vi "MGCC_MdlMgmt_others.vi"() -> ()   [LabVIEW 2016]
doc: "This VI is designed to initize the SHE215 model with Slack, NumN, NumL, NumC, NumZ, NumR and NumS (double)."
panel:
  out "text":string
  out "array":dbl[](array[numeric])
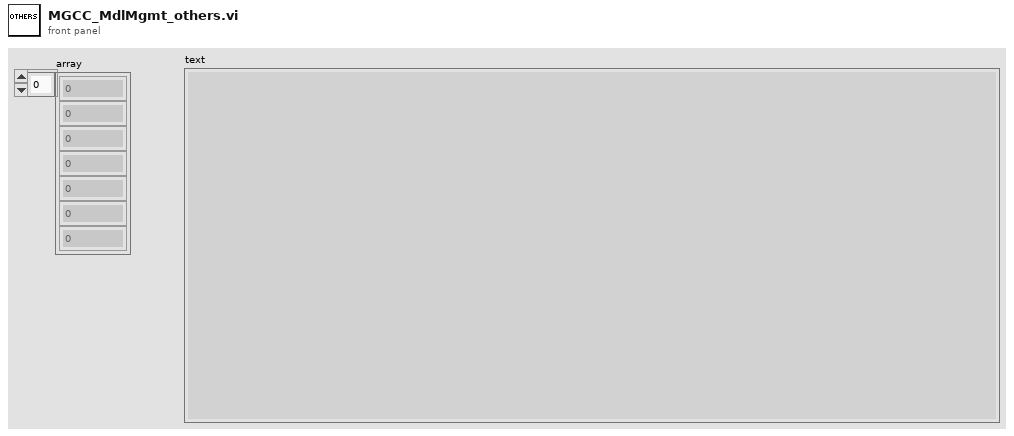
[diagram p1: front panel]
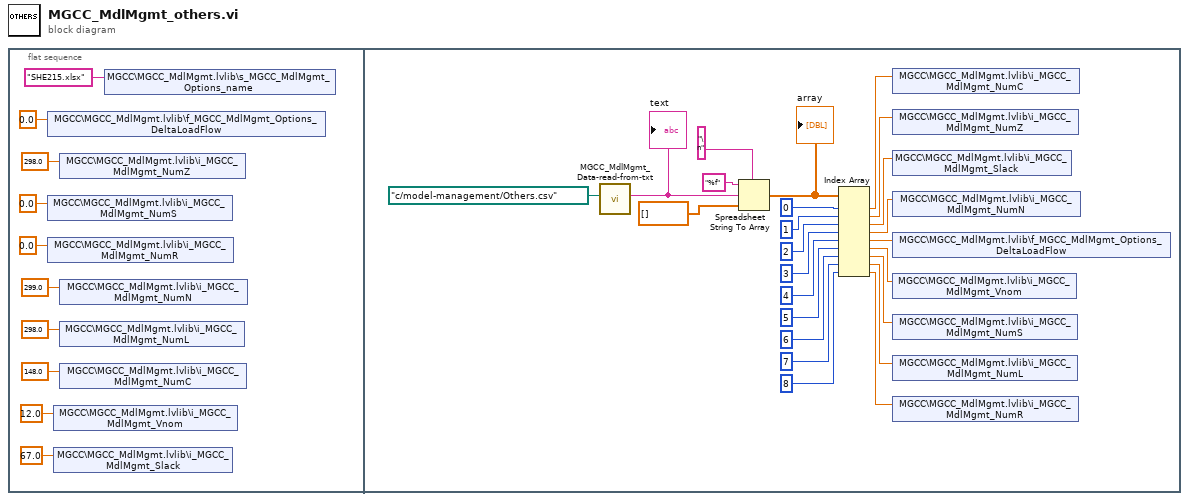
[diagram p0: block diagram]
diagram:
  n1 = flat-sequence {
    frame #0 {
      n2 = shared-variable "MGCC\\MGCC_MdlMgmt.lvlib\\f_MGCC_MdlMgmt_Options_DeltaLoadFlow"(0.0 ("MGCC_MdlMgmt_Options_DeltaLoadFlow")) -> ()  [unwired: 1 in, 1 out]
      n3 = shared-variable "MGCC\\MGCC_MdlMgmt.lvlib\\i_MGCC_MdlMgmt_NumS"(0.0 ("MGCC_MdlMgmt_NumS")) -> ()  [unwired: 1 in, 1 out]
      n4 = shared-variable "MGCC\\MGCC_MdlMgmt.lvlib\\i_MGCC_MdlMgmt_NumR"(0.0 ("MGCC_MdlMgmt_NumR")) -> ()  [unwired: 1 in, 1 out]
      n5 = shared-variable "MGCC\\MGCC_MdlMgmt.lvlib\\i_MGCC_MdlMgmt_Vnom"(12.0 ("MGCC_MdlMgmt_Vnom")) -> ()  [unwired: 1 in, 1 out]
      n6 = shared-variable "MGCC\\MGCC_MdlMgmt.lvlib\\i_MGCC_MdlMgmt_Slack"(67.0 ("MGCC_MdlMgmt_Slack")) -> ()  [unwired: 1 in, 1 out]
      n7 = shared-variable "MGCC\\MGCC_MdlMgmt.lvlib\\i_MGCC_MdlMgmt_NumZ"(298.0 ("MGCC_MdlMgmt_NumZ")) -> ()  [unwired: 1 in, 1 out]
      n8 = shared-variable "MGCC\\MGCC_MdlMgmt.lvlib\\i_MGCC_MdlMgmt_NumN"(299.0 ("MGCC_MdlMgmt_NumN")) -> ()  [unwired: 1 in, 1 out]
      n9 = shared-variable "MGCC\\MGCC_MdlMgmt.lvlib\\i_MGCC_MdlMgmt_NumL"(298.0 ("MGCC_MdlMgmt_NumL")) -> ()  [unwired: 1 in, 1 out]
      n10 = shared-variable "MGCC\\MGCC_MdlMgmt.lvlib\\i_MGCC_MdlMgmt_NumC"(148.0 ("MGCC_MdlMgmt_NumC")) -> ()  [unwired: 1 in, 1 out]
      n11 = shared-variable "MGCC\\MGCC_MdlMgmt.lvlib\\s_MGCC_MdlMgmt_Options_name"("SHE215.xlsx" ("MGCC_MdlMgmt_Options_name")) -> ()  [unwired: 1 in, 1 out]
    }
    frame #1 {
      n12 = call "MGCC_MdlMgmt_Data-read-from-txt.vi"("file path (use dialog)"=path "c:/model-management/Others.csv") -> ("text"=w31:string)  [unwired: 10 in]
      "text" <- w31
      n13 = Spreadsheet String To Array(delimiter (Tab)="\n", format string="%f", spreadsheet string=w31, array type (2D Dbl)=dbl[] []) -> (array=w30:dbl[])
      "array" <- w30
      n14 = Index Array(array=w30, index #1=0 ("index"), index #2=1 ("index"), index #3=2 ("index"), index #4=3 ("index"), index #5=4 ("index"), index #6=5 ("index"), index #7=6 ("index"), index #8=7 ("index"), index #9=8 ("index")) -> (element #1=w20:dbl, element #2=w19:dbl, element #3=w18:dbl, element #4=w17:dbl, element #5=w16:dbl, element #6=w15:dbl, element #7=w14:dbl, element #8=w13:dbl, element #9=w12:dbl)
      n15 = shared-variable "MGCC\\MGCC_MdlMgmt.lvlib\\i_MGCC_MdlMgmt_NumC"(w20) -> ()  [unwired: 1 in, 1 out]
      n16 = shared-variable "MGCC\\MGCC_MdlMgmt.lvlib\\i_MGCC_MdlMgmt_NumZ"(w19) -> ()  [unwired: 1 in, 1 out]
      n17 = shared-variable "MGCC\\MGCC_MdlMgmt.lvlib\\i_MGCC_MdlMgmt_Slack"(w18) -> ()  [unwired: 1 in, 1 out]
      n18 = shared-variable "MGCC\\MGCC_MdlMgmt.lvlib\\i_MGCC_MdlMgmt_NumN"(w17) -> ()  [unwired: 1 in, 1 out]
      n19 = shared-variable "MGCC\\MGCC_MdlMgmt.lvlib\\f_MGCC_MdlMgmt_Options_DeltaLoadFlow"(w16) -> ()  [unwired: 1 in, 1 out]
      n20 = shared-variable "MGCC\\MGCC_MdlMgmt.lvlib\\i_MGCC_MdlMgmt_Vnom"(w15) -> ()  [unwired: 1 in, 1 out]
      n21 = shared-variable "MGCC\\MGCC_MdlMgmt.lvlib\\i_MGCC_MdlMgmt_NumS"(w14) -> ()  [unwired: 1 in, 1 out]
      n22 = shared-variable "MGCC\\MGCC_MdlMgmt.lvlib\\i_MGCC_MdlMgmt_NumL"(w13) -> ()  [unwired: 1 in, 1 out]
      n23 = shared-variable "MGCC\\MGCC_MdlMgmt.lvlib\\i_MGCC_MdlMgmt_NumR"(w12) -> ()  [unwired: 1 in, 1 out]
    }
  }
